vi "Read Latest Broadcast.vi"(8 "error in (no error)":errorcluster, 11 "Debug Latest Message in":refnum<class "Debug Latest Broadcast.lvclass">) -> (0 "error out":errorcluster, 2 "Latest Messages":map{string, refnum<class "Debug Data.lvclass">}(c390), 3 "Debug Latest Message out":refnum<class "Debug Latest Broadcast.lvclass">)   [LabVIEW 2020, in "Debug Latest Broadcast.lvclass"]
uses:
  Debug Latest Broadcast.lvclass
  Debug Data/Debug Data.lvclass
  Debug Latest Broadcast.lvclass/Debug Latest Broadcast.ctl
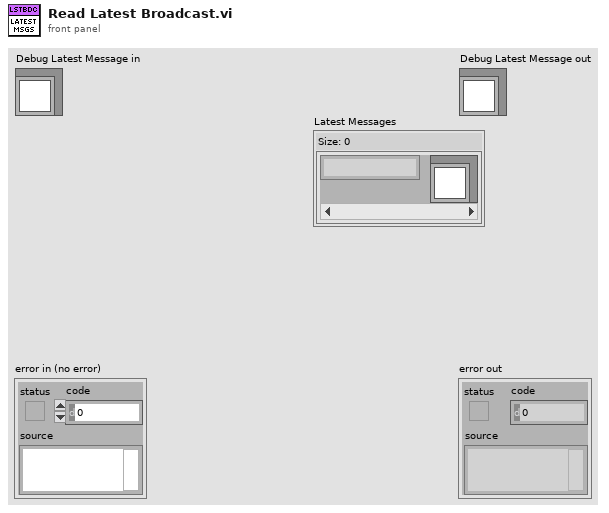
[diagram p1: front panel]
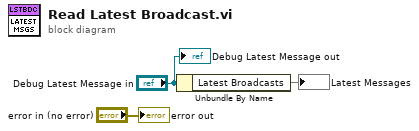
[diagram p0: block diagram]
diagram:
  n1 = Unbundle By Name("Debug Latest Message in") -> ("Latest Broadcasts"=→"Latest Messages":map{string, refnum<class "Debug Data.lvclass">})
  "error out" <- "error in (no error)"
  "Debug Latest Message out" <- "Debug Latest Message in"
